vi "Create.vi"(8 "error in (no error)":errorcluster, 9 "Path":string, 10 "Label":string) -> (0 "error out":errorcluster, 3 "Nav Route out":refnum<class "Nav Route.lvclass">)   [LabVIEW 2020, in "Volatus.lvlib" / "Nav Route.lvclass"]
uses:
  Nav Route.lvclass
  Nav Route.lvclass/Nav Route.ctl
  lv-exec-anchor/ExecAnchor/ExecAnchor.lvclass
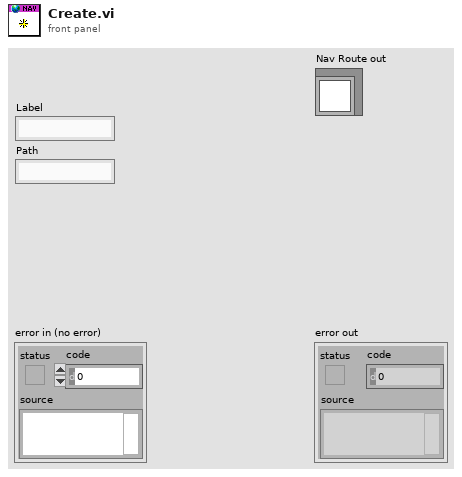
[diagram p1: front panel]
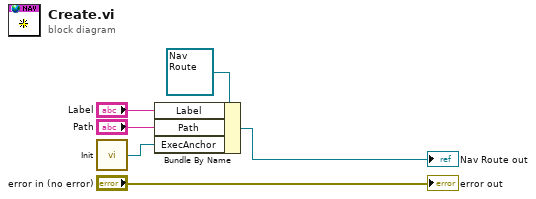
[diagram p0: block diagram]
diagram:
  n1 = call "Init.vi"() -> ("ExecAnchor out"=w1:refnum<class "ExecAnchor.lvclass">)  [unwired: 7 in]
  n2 = Bundle By Name(cluster=refnum<class "Nav Route.lvclass"> refnum ("Nav Route in"), "Label"="Label", "Path"="Path", "ExecAnchor"=w1) -> (→"Nav Route out":refnum<class "Nav Route.lvclass">)
  "error out" <- "error in (no error)"
